vi "Get Job File Counts.vi"(8 "error in":errorcluster, 11 "Job Folder":path) -> (0 "error out":errorcluster, 1 "Produced Count":i32, 2 "Consumed Count":i32)   [LabVIEW 2015]
doc: "This vi is used to find the read the input file and output file count from the modeler configuration file for the job\n\nInputs\nThe job folder path\nThe extension of the configuration file\nThe section name for the files configuration\nThe consumed count field name\nThe producted count field name\n\nOutputs\nConsumed count (needed by the modeler as inputs)\nProduced count (created by the modeler at completion)"
panel:
  in  "Section":string="FileConfiguration"
  in  "Produced Count Field Name":string="Produced"
  in  "Consumed Count Field Name":string="Consumed"
  in  "Config.ext":string="xml"
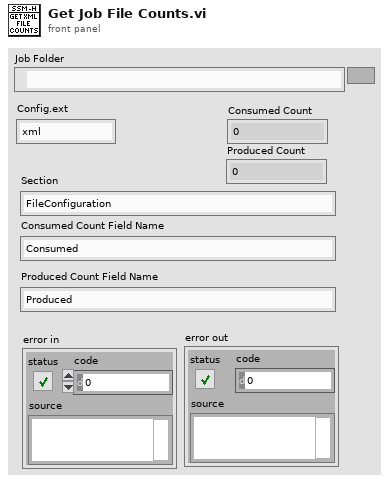
[diagram p1: front panel]
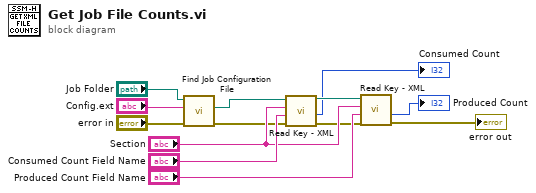
[diagram p0: block diagram]
diagram:
  n1 = call "Find Job Configuration File.vi"("error in (no error)"="error in", "Config.ext"="Config.ext", "Job Folder"="Job Folder") -> ("error out"=w4:errorcluster, "Config File"=w2:path)  [unwired: 6 in, 1 out]
  n2 = call "Read Key - XML.vi"("error in (no error)"=w4, "Key"="Consumed Count Field Name", "Section"="Section", "XML file"=w2) -> ("error out"=w7:errorcluster, "Value Number"=→"Consumed Count":i32, "XML file out"=w6:path)  [unwired: 4 in, 1 out]
  n3 = call "Read Key - XML.vi"("error in (no error)"=w7, "Key"="Produced Count Field Name", "Section"="Section", "XML file"=w6) -> ("error out"=→"error out":errorcluster, "Value Number"=→"Produced Count":i32)  [unwired: 4 in, 2 out]
